vi "GenerateData.vi"() -> ()   [LabVIEW 2017]
uses:
  GlobalVariable.vi
panel:
  out "error out":errorcluster
  in  "stop":bool
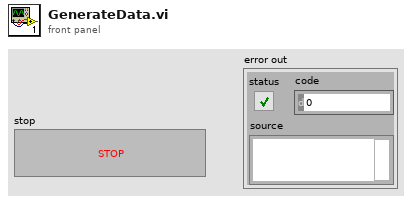
[diagram p1: front panel]
types:
  T1 = enum16{"open", "replace", "create", "open or create", "replace or create", "replace or create with confirmation"}
  T2 = typedef "Semaphore RefNum" = refnum<k1>
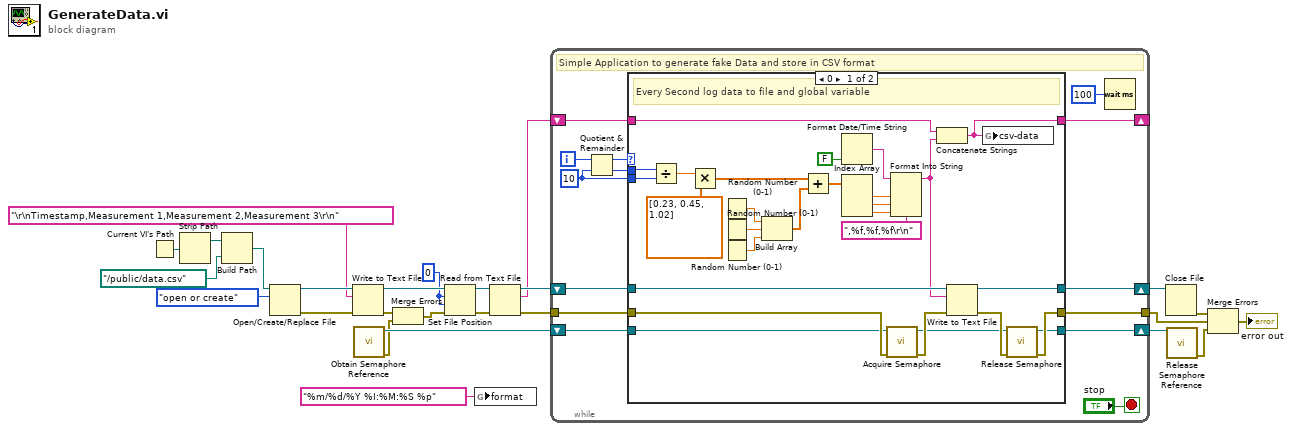
[diagram p0: block diagram]
diagram:
  w2 = i64 0 ("offset (in bytes) (0)")
  n1 = Current VI's Path() -> (path=w21:path)
  n2 = Strip Path(path=w21) -> (stripped path=w20:path)  [unwired: 1 out]
  n3 = Build Path(base path=w20, name or relative path=path "../public/data.csv" ("file path (use dialog)")) -> (appended path=w18:path)
  n4 = Open/Create/Replace File(file path (use dialog)=w18, operation (0:open)=T1."open or create") -> (refnum out=w16:refnum<file>, error out=w17:errorcluster)  [unwired: 4 in, 1 out]
  n5 = Write to Text File(file (use dialog)=w16, text="\r\nTimestamp,Measurement 1,Measurement 2,Measurement 3\r\n", error in=w17) -> (refnum out=w6:refnum<file>, error out=w11:errorcluster)  [unwired: 1 in, 1 out]
  n6 = call <vilib>:"Obtain Semaphore Reference.vi"() -> ("error out"=w10:errorcluster, "semaphore"=w12:T2)  [unwired: 5 in, 1 out]
  n7 = Merge Errors(w11, w10) -> (w5:errorcluster)
  n8 = Set File Position(offset (in bytes) (0)=w2, refnum=w6, from (0:start)=w2, error in=w5) -> (refnum out=w3:refnum<file>, error out=w4:errorcluster)
  n9 = global write "GlobalVariable.vi" "format"("%m/%d/%Y %I:%M:%S %p") -> ()
  n10 = Read from Text File(file (use dialog)=w3, error in=w4) -> (refnum out=w9:refnum<file>, text=w7:string, error out=w8:errorcluster)  [unwired: 2 in, 1 out]
  n11 = while {
    tunnel: w8 -> [w36]
    tunnel: [w35] -> w25
    shift-right: [w34] -> w26
    shift-left: w9 -> [w33]
    shift-right: [w30] -> w14
    shift-left: w12 -> [w29]
    shift-right: [w27] -> _
    shift-left: w7 -> [w28]
    i -> [w37]
    stop <- "stop" stop-if-true
    w32 = 10 ("y")
    # "Simple Application to generate fake Data and store in CSV format"
    n12 = Quotient & Remainder(x=w37, y=w32) -> (x-y*floor(x/y)=w38:i32, floor(x/y)=w31:i32)
    n13 = case shown="0" w38 {
      tunnel: w36 -> [w47 w72]
      tunnel: [w49 w72] -> w35
      tunnel: [w67 w71] -> w34
      tunnel: w33 -> [w68 w71]
      tunnel: w32 -> [w66 _]
      tunnel: w31 -> [w64 _]
      tunnel: [w48 w70] -> w30
      tunnel: w29 -> [w44 w70]
      tunnel: w28 -> [w43 w69]
      tunnel: [w41 w69] -> w27
      frame 0 {
        # "Every Second log data to file and global variable"
        n14 = Divide(x=w64, y=w66) -> (x/y=w53:dbl)
        n15 = Multiply(x=w53, y=dbl[] [0.23, 0.45, 1.02]) -> (x*y=w52:dbl[])
        n16 = Random Number (0-1)() -> (number: 0 to 1=w59:dbl)
        n17 = Random Number (0-1)() -> (number: 0 to 1=w60:dbl)
        n18 = Random Number (0-1)() -> (number: 0 to 1=w58:dbl)
        n19 = Build Array(w59, w60, w58) -> (w61:dbl[])
        n20 = Add(x=w52, y=w61) -> (x+y=w54:dbl[])
        n21 = Format Date/Time String(UTC format=FALSE) -> (date/time string=w62:string)  [unwired: 2 in]
        n22 = Index Array(array=w54) -> (element #1=w57:dbl, element #2=w56:dbl, element #3=w55:dbl)  [unwired: 3 in]
        n23 = call <vilib>:"Acquire Semaphore.vi"("error in (no error)"=w47, "semaphore"=w44) -> ("error out"=w46:errorcluster, "semaphore out"=w45:T2)  [unwired: 3 in, 1 out]
        n24 = Format Into String(format string=",%f,%f,%f\r\n", initial string=w62, w57, w56, w55) -> (resulting string=w42:string)  [unwired: 1 in, 1 out]
        n25 = Concatenate Strings(w43, w42) -> (w41:string)
        n26 = Write to Text File(file (use dialog)=w68, text=w42, error in=w46) -> (refnum out=w67:refnum<file>, error out=w50:errorcluster)  [unwired: 1 in, 1 out]
        n27 = global write "GlobalVariable.vi" "csv-data"(w41) -> ()
        n28 = call <vilib>:"Release Semaphore.vi"("error in (no error)"=w50, "semaphore"=w45) -> ("error out"=w49:errorcluster, "semaphore out"=w48:T2)  [unwired: 4 in]
      }
      frame Default {
      }
    }
    n29 = Wait (ms)(milliseconds to wait=u32 100) -> ()  [unwired: 1 out]
  }
  n30 = Close File(refnum=w26) -> (error out=w24:errorcluster)  [unwired: 1 in, 1 out]
  n31 = call <vilib>:"Release Semaphore Reference.vi"("semaphore"=w14) -> ("error out"=w13:errorcluster)  [unwired: 9 in, 1 out]
  n32 = Merge Errors(w24, w25, w13) -> (→"error out":errorcluster)
